vi "StageMotion.vi"() -> ()   [LabVIEW 2016]
uses:
  <vilib>/Utility/file.llb/Write Delimited Spreadsheet (DBL).vi
panel:
  in  "X Shifts [mm]":dbl[](array[numeric])=[90.0, 180.0, 270.0]
  in  "Cycles":i32=50
  out "Running Times [s]":dbl[](array[numeric])
  in  "Times [s]":dbl[](array[numeric])
  in  "Start [mm]":dbl[](array[numeric])=[100.0, 0.0, -10.0]
  in  "Axis Speeds [mm/s]":T1={"X [mm/s]"=15.0, "Y [mm/s]"=15.0, "Z [mm/s]"=15.0}
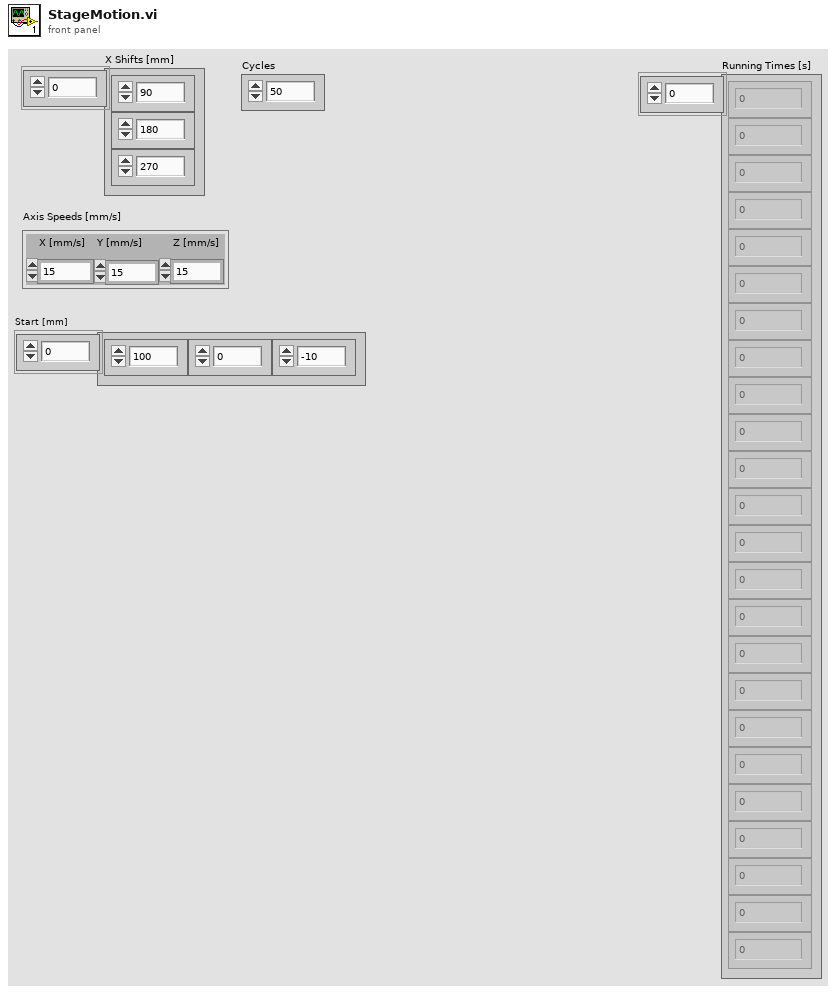
[diagram p1: front panel]
types:
  T1 = cluster{"X [mm/s]":dbl, "Y [mm/s]":dbl, "Z [mm/s]":dbl}
  T2 = cluster{"Start [mm][0]":dbl, "Start [mm][1]":dbl, "Start [mm][2]":dbl}
  T3 = cluster{"Final X":dbl, "Final Y":dbl, "Final Z":dbl}
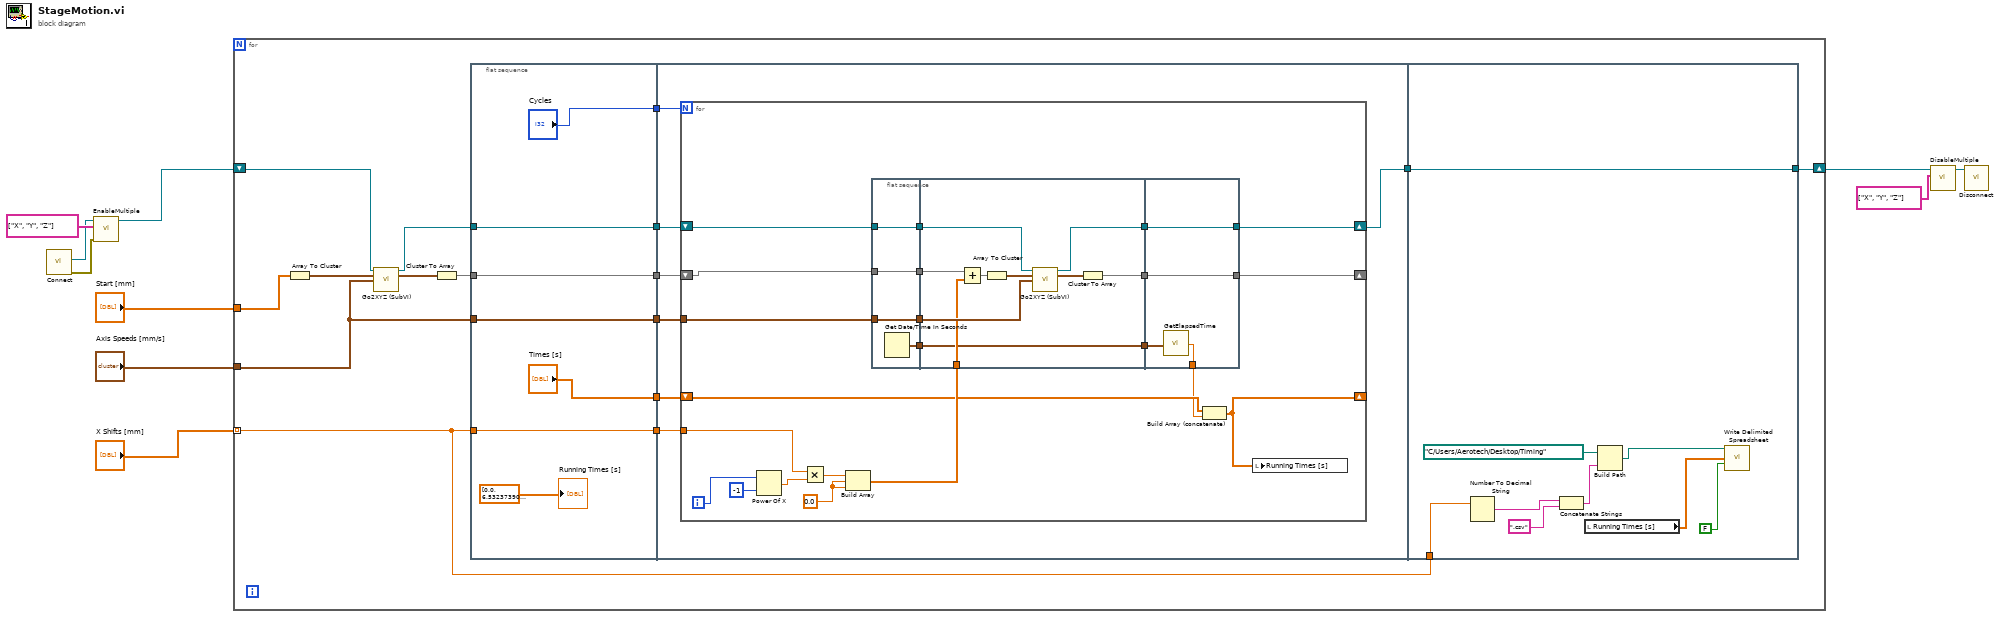
[diagram p0: block diagram]
diagram:
  n1 = call "Connect.vi"() -> ("error out"=w8:errorcluster, "controller"=w9:refnum<k24>)  [unwired: 10 in]
  n2 = call "EnableMultiple.vi"("error in (no error)"=w8, "axis names"=string[] ["X", "Y", "Z"] ("Axes Names"), "controller in"=w9) -> ("controller out"=w6:refnum<k24>)  [unwired: 7 in, 1 out]
  n3 = for {
    tunnel: "Start [mm]" -> [w25]
    tunnel: "Axis Speeds [mm/s]" -> [w20]
    shift-right: [w19] -> w2
    shift-left: w6 -> [w21]
    tunnel: "X Shifts [mm]" -> [w11] mode=indexing
    n4 = Array To Cluster(array=w25) -> (cluster=w26:T2)
    n5 = call "Go2XYZ (SubVI).vi"(".NET Refnum in"=w21, "Go to Coordinates"=w26, "Axis Speeds"=w20) -> (".NET Refnum out"=w22:refnum<k24>, "Final Position"=w24:T3)  [unwired: 8 in, 3 out]
    n6 = Cluster To Array(cluster=w24) -> (array=w23:dbl[])
    n7 = flat-sequence {
      tunnel: w11 -> [w30]
      tunnel: w20 -> [w31]
      tunnel: w22 -> [w32]
      tunnel: w23 -> [w33]
      tunnel: [w33] -> w18
      tunnel: [w32] -> w17
      tunnel: [w31] -> w16
      tunnel: [w30] -> w15
      tunnel: ["Cycles"] -> w14
      tunnel: ["Times [s]"] -> w13
      tunnel: w18 -> [w40]
      tunnel: w17 -> [w39]
      tunnel: w16 -> [w38]
      tunnel: w15 -> [w36]
      tunnel: w14 -> [w35]
      tunnel: w13 -> [w34]
      tunnel: [w37] -> w12
      tunnel: [w89] -> w19
      tunnel: w12 -> [w89]
      tunnel: w11 -> [w87]
      frame #0 {
        "Running Times [s]" <- dbl[] [0.0, 6.532373905181885, 6.490371227264404, 6.40536642074585, 6.4043660163879395, 6.2733588218688965, 6.179353713989258, 6.4043660163879395, 6.404366493225098, 6.247357368469238, 6.4073662757873535, 6.341362953186035, 6.203354835510254, 6.538373947143555, 6.276358604431152, 6.532373905181885, 6.4023661613464355, 6.464369773864746, 6.348362922668457, 6.536374092102051, 6.406366348266602, 6.170352935791016, 6.177353382110596, 6.1793532371521, 6.338362693786621, 6.235356330871582, 6.403366565704346, 6.177353382110596, 6.291359901428223, 6.405365943908691, 6.16735315322876, 6.244357109069824, 6.406366348266602, 6.409366607666016, 6.2693586349487305, 6.401366233825684, 6.174353122711182, 6.245357036590576, 6.401366233825684, 6.351363182067871, 6.463369846343994, 6.4043660163879395, 6.362364292144775, 6.246356964111328, 6.247357368469238, 6.3783650398254395, 6.251357078552246, 6.537374019622803, 6.513372898101807, 6.353363037109375, 6.409366607666016, 6.388365745544434, 6.244357109069824, 6.400365829467773, 6.40536642074585, 6.205355167388916, 6.4023661613464355, 6.266358375549316, 6.17335319519043, 6.208354949951172, 6.250357627868652, 6.1723527908325195, 6.408366680145264, 6.40536642074585, 6.5293731689453125, 6.312361240386963, 6.404366493225098, 6.334362030029297, 6.170352935791016, 6.401366233825684, 6.177353382110596, 6.24835729598999, 6.404366493225098, 6.225356101989746, 6.40536642074585, 6.201354503631592, 6.411366939544678, 6.211355209350586, 6.401366233825684, 6.1853532791137695, 6.24235725402832, 6.401366233825684, 6.490371227264404, 6.240356922149658, 6.4073662757873535, 6.290359973907471, 6.240356922149658, 6.404366493225098, 6.2903594970703125, 6.2723588943481445, 6.4043660163879395, 6.18735408782959, 6.400366306304932, 6.406366348266602, 6.247357368469238, 6.4043660163879395, 6.407366752624512, 6.384365081787109, 6.24135684967041, 6.172353267669678] ("Running Times [s]")
      }
      frame #1 {
        n8 = for {
          N: w35 -> [_]
          shift-right: [w52] -> _
          shift-left: w40 -> [w54]
          shift-right: [w59] -> w37
          shift-left: w39 -> [w60]
          tunnel: w38 -> [w55]
          shift-right: [w41] -> _
          shift-left: w34 -> [w44]
          tunnel: w36 -> [w42]
          i -> [w62]
          w56 = 0.0 ("element")
          n9 = Power Of X(1:-1 ("x"), 2:w62) -> (0:w58:dbl)
          n10 = Multiply(x=w42, y=w58) -> (x*y=w57:dbl)
          n11 = Build Array(w57, w56, w56) -> (w53:dbl[])
          n12 = flat-sequence {
            tunnel: w54 -> [w64]
            tunnel: w55 -> [w65]
            tunnel: w60 -> [w66]
            tunnel: [w66] -> w49
            tunnel: [w65] -> w48
            tunnel: [w64] -> w47
            tunnel: [w63] -> w46
            tunnel: w53 -> [w70]
            tunnel: [w75] -> w51
            tunnel: [w68] -> w50
            tunnel: w49 -> [w76]
            tunnel: w48 -> [w73]
            tunnel: w47 -> [w72]
            tunnel: w46 -> [w67]
            tunnel: [w67] -> w45
            tunnel: [w79] -> w52
            tunnel: [w80] -> w59
            tunnel: w51 -> [w80]
            tunnel: w50 -> [w79]
            tunnel: w45 -> [w78]
            tunnel: [w77] -> w43
            frame #0 {
              n13 = Get Date/Time In Seconds() -> (seconds since 1Jan1904=w63:timestamp)
            }
            frame #1 {
              n14 = Add(x=w72, y=w70) -> (x+y=w71:dbl[])
              n15 = Array To Cluster(array=w71) -> (cluster=w74:cluster{"[0]":dbl, "[1]":dbl, "[2]":dbl})
              n16 = call "Go2XYZ (SubVI).vi"(".NET Refnum in"=w76, "Go to Coordinates"=w74, "Axis Speeds"=w73) -> (".NET Refnum out"=w75:refnum<k24>, "Final Position"=w69:T3)  [unwired: 8 in, 3 out]
              n17 = Cluster To Array(cluster=w69) -> (array=w68:dbl[])
            }
            frame #2 {
              n18 = call "GetElapsedTime.vi"("Start Time"=w78) -> ("Elapsed Time [s]"=w77:sgl)
            }
          }
          n19 = Build Array (concatenate)(w44, w43) -> (w41:dbl[])
          n20 = local write "Running Times [s]"(w41) -> ()
        }
      }
      frame #2 {
        n21 = Number To Decimal String(number=w87) -> (decimal integer string=w86:string)  [unwired: 1 in]
        n22 = Concatenate Strings(w86, ".csv" ("string")) -> (w85:string)
        n23 = local read "Running Times [s]"() -> (w82:dbl[])
        n24 = Build Path(base path=path "C:/Users/Aerotech/Desktop/Timing", name or relative path=w85) -> (appended path=w83:path)
        n25 = call-poly <vilib>:"Write Delimited Spreadsheet.vi"("file path (dialog if empty)"=w83, "1D data"=w82, "append to file? (new file:F)"=FALSE) -> ()  [unwired: 11 in, 2 out]
      }
    }
  }
  n26 = call "DisableMultiple.vi"("axis names"=string[] ["X", "Y", "Z"], "controller in"=w2) -> ("controller out"=w4:refnum<k24>)  [unwired: 8 in, 1 out]
  n27 = call "Disconnect.vi"("controller"=w4) -> ()  [unwired: 10 in, 1 out]
